vi "close.vi"(8 "error in":errorcluster, 10 "data":variant) -> (0 "error out":errorcluster)   [LabVIEW 2018, in "Entry Console.lvlib"]
doc: "This VI enqueues the named action"
uses:
  Entry Console.lvlib
  Private Controls/Module Data Cluster.ctl
  Private Controls/Module Action.ctl
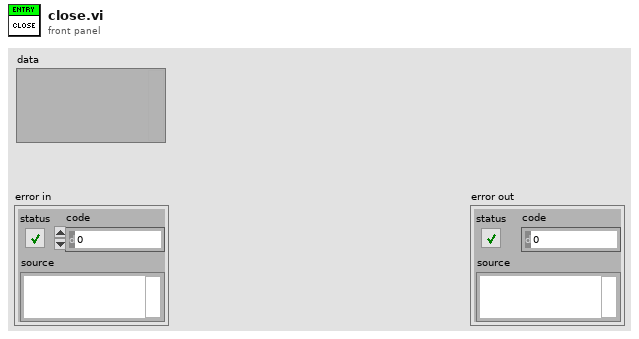
[diagram p1: front panel]
types:
  T1 = typedef "Entry Console.lvlib/Module Data Cluster.ctl" = cluster{"Variant":variant, "action":T2}
  T2 = typedef "Entry Console.lvlib/Module Action.ctl" = enum16{"error", "exit", "Start Wash", "init", "Enable Wash Buttons"}
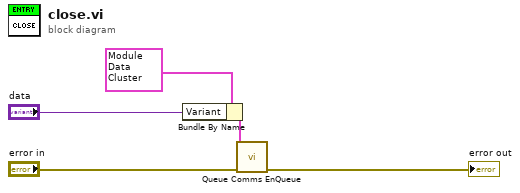
[diagram p0: block diagram]
diagram:
  n1 = Bundle By Name(cluster=T1 {"Variant"=variant, "action"=enum."error"} ("Module Data Cluster"), "Variant"="data") -> (w4:T1)
  n2 = call "Queue Comms EnQueue.vi"("error in"="error in", "Module Data Cluster"=w4) -> ("error out"=→"error out":errorcluster)  [unwired: 9 in]
